vi "Cooler Test.vi"() -> ()   [LabVIEW 2012]
uses:
  <vilib>/ActorFramework/Actor/Actor.lvclass
  <vilib>/ActorFramework/Stop Msg/Stop Msg.lvclass
  Level Controller/Level Controller/Level Controller.lvclass
  Cooler/Cooler/Cooler.lvclass
  <vilib>/ActorFramework/Message Queue/Message Queue.lvclass
  Level Controller/Level Controller Messages/Write Deadband Msg/Write Deadband Msg.lvclass
panel:
  in  "Set Point":dbl=75.0
  in  "stop":bool
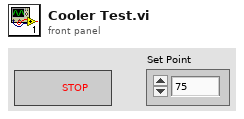
[diagram p1: front panel]
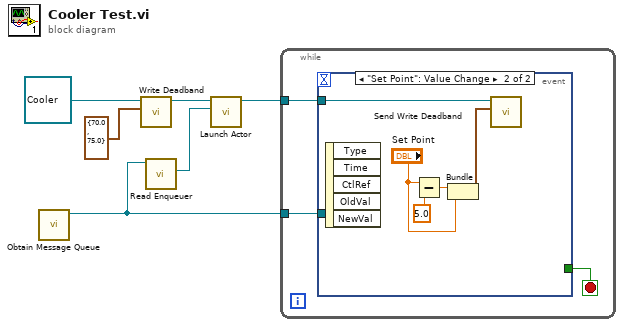
[diagram p0: block diagram]
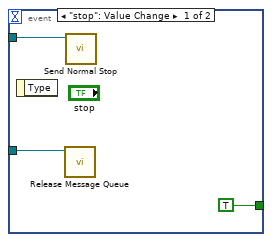
[diagram p2: hidden frame]
diagram:
  n1 = call <vilib>:"Obtain Message Queue.vi"() -> ("Message Queue"=w6:refnum<class "Message Queue.lvclass">)  [unwired: 10 in, 1 out]
  n2 = call "Write Deadband.vi"("Deadband"=cluster{"LO":dbl, "HI":dbl} {"LO"=70.0, "HI"=75.0}, "Level Controller in"=refnum<class "Cooler.lvclass"> refnum ("Cooler.lvlib:Cooler.lvclass")) -> ("Level Controller out"=w3:refnum<class "Level Controller.lvclass">)  [unwired: 8 in, 1 out]
  n3 = call <vilib>:"Read Enqueuer.vi"("Message Queue"=w6) -> ("Message Enqueuer"=w4:refnum<class "Message Enqueuer.lvclass">)  [unwired: 10 in]
  n4 = call <vilib>:"Launch Actor.vi"("Actor-to-Caller Enqueuer"=w4, "Actor"=w3) -> ("Caller-To-Actor Enqueuer"=w5:refnum<class "Message Enqueuer.lvclass">)  [unwired: 8 in, 1 out]
  n5 = while {
    tunnel: w6 -> [w9]
    tunnel: w5 -> [w8]
    stop <- w7 stop-if-true
    n6 = event shown="[1] \"Set Point\": Value Change" {
      selector: _ -> [_ _]
      dyn-events: _ -> [_ _]
      timeout: _ -> [_ _]
      tunnel: w8 -> [w12 w14]
      tunnel: w9 -> [w11 _]
      tunnel: [TRUE _] -> w7
      event "stop": Value Change {
        n7 = event-data() -> ()  [unwired: 1 in, 1 out]
        n8 = call <vilib>:"Release Message Queue.vi"("Message Queue"=w11) -> ()  [unwired: 9 in, 2 out]
        n9 = call <vilib>:"Send Normal Stop.vi"("Message Enqueuer"=w12) -> ()  [unwired: 10 in, 1 out]
      }
      event "Set Point": Value Change {
        n10 = event-data() -> ()  [unwired: 1 in, 5 out]
        n11 = Subtract(x="Set Point", y=5.0) -> (x-y=w16:dbl)
        n12 = Bundle(w16, "Set Point"="Set Point") -> (w13:cluster{dbl, "Set Point":dbl})  [unwired: 1 in]
        n13 = call "Send Write Deadband.vi"("Deadband"=w13, "Message Enqueuer"=w14) -> ()  [unwired: 8 in, 2 out]
      }
    }
  }
